vi "FindElementStartByNameC.vi"(6 "offset (0)":i32, 10 "Element Name":string, 11 "string":string) -> (1 "after substring":string, 2 "match substring":string, 3 "before substring":string, 4 "offset past match":i32)   [LabVIEW 2017]
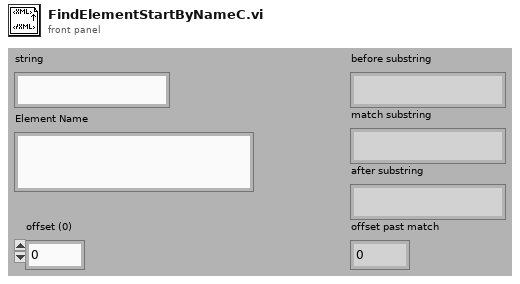
[diagram p1: front panel]
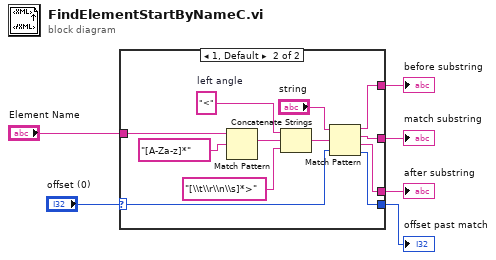
[diagram p0: block diagram]
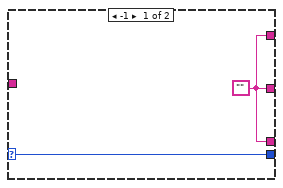
[diagram p2: hidden frame]
diagram:
  n1 = case shown="1, Default" "offset (0)" {
    selector: "offset (0)" -> [w8 w13]
    tunnel: [w7 w17] -> w6
    tunnel: [w7 w16] -> w5
    tunnel: [w8 w15] -> w4
    tunnel: [w7 w14] -> w3
    tunnel: "Element Name" -> [_ w11]
    frame -1 {
      w7 = ""
    }
    frame 1, Default {
      w20 = "<"  # left angle
      n2 = Match Pattern(string=w11, regular expression="[A-Za-z]*") -> (match substring=w10:string)  [unwired: 1 in, 3 out]
      n3 = Concatenate Strings(w20, w10, "[\\t\\r\\n\\s]*>" ("regular expression")) -> (w18:string)
      n4 = Match Pattern(string="string", regular expression=w18, offset (0)=w13) -> (before substring=w17:string, match substring=w14:string, after substring=w16:string, offset past match=w15:i32)
    }
  }
  "before substring" <- w6
  "match substring" <- w3
  "after substring" <- w5
  "offset past match" <- w4
